vi "start.vi"(8 "error in (no error)":errorcluster, 11 "Model in":refnum<class "Model.lvclass">) -> (0 "error out":errorcluster, 3 "Model out":refnum<class "Model.lvclass">)   [LabVIEW 2013, in "Model.lvclass"]
uses:
  Model.lvclass
  Model.lvclass/Model.ctl
  <userlib>/Common/ILC/ILC/ILC.lvclass
  <userlib>/Common/Component/Application/Application/Application.lvclass
  ConfigurationThisComponent/ConfigurationThisComponent.lvclass
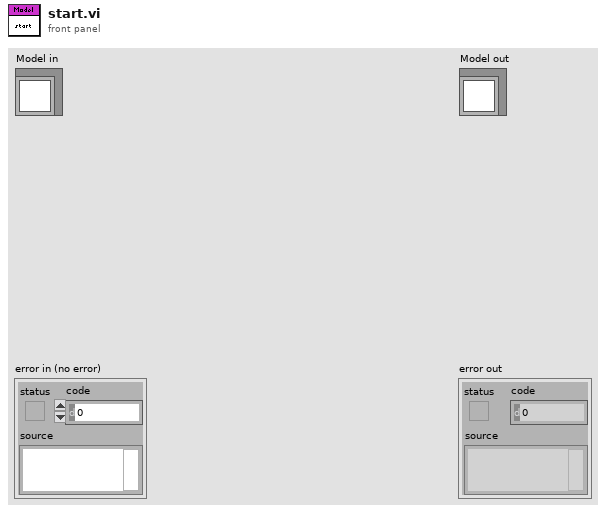
[diagram p1: front panel]
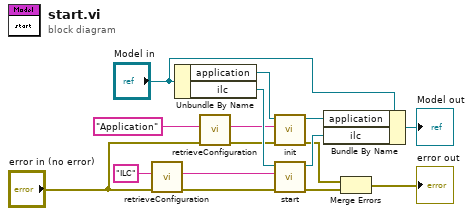
[diagram p0: block diagram]
diagram:
  n1 = call "retrieveConfiguration.vi"("error in (no error)"="error in (no error)", "configName"="ILC") -> ("error out"=w5:errorcluster, "xmlConfig"=w7:string)  [unwired: 7 in, 1 out]
  n2 = Unbundle By Name("Model in") -> ("application"=w12:refnum<class "Application.lvclass">, "ilc"=w14:refnum<class "ILC.lvclass">)
  n3 = call "retrieveConfiguration.vi"("error in (no error)"="error in (no error)", "configName"="Application") -> ("error out"=w4:errorcluster, "xmlConfig"=w8:string)  [unwired: 7 in, 1 out]
  n4 = call <userlib>:"init.vi"("error in (no error)"=w4, "xmlConfig"=w8, "Application in"=w12) -> ("error out"=w3:errorcluster, "Application out"=w11:refnum<class "Application.lvclass">)  [unwired: 7 in]
  n5 = call <userlib>:"start.vi"("error in (no error)"=w5, "xmlConfig"=w7, "ILC in"=w14) -> ("error out"=w2:errorcluster, "ILC out"=w13:refnum<class "ILC.lvclass">)  [unwired: 7 in]
  n6 = Bundle By Name(cluster="Model in", "application"=w11, "ilc"=w13) -> (→"Model out":refnum<class "Model.lvclass">)
  n7 = Merge Errors(w3, w2) -> (→"error out":errorcluster)
